vi "Get Sheet List.vi"(8 "error in (no error)":errorcluster, 11 "MS-Excel in":refnum<class "MS-Excel.lvclass">) -> (0 "error out":errorcluster, 2 "Sheet List":string[](array[string]), 3 "MS-Excel out":refnum<class "MS-Excel.lvclass">)   [LabVIEW 2017, in "LabVIEW NPOI.lvlib" / "MS-Excel.lvclass"]
doc: "Returns the names list, in <b>Sheet List</b>, of worksheets into the associated workbook to the <b>Document</b>."
uses:
  MS-Excel.lvclass
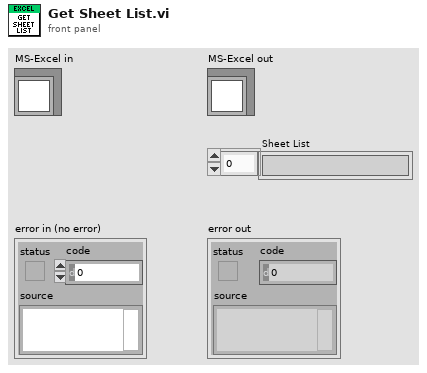
[diagram p1: front panel]
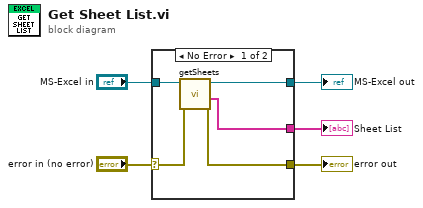
[diagram p0: block diagram]
diagram:
  n1 = case shown="No Error" "error in (no error)" {
    selector: "error in (no error)" -> [w8 w12]
    tunnel: [w7 w12] -> w4
    tunnel: [w9 w11] -> w2
    tunnel: "MS-Excel in" -> [w10 w11]
    tunnel: [w6 _] -> w1
    frame No Error {
      n2 = call-dynamic "getSheets.vi"("error in (no error)"=w8, "MS-Excel in"=w10) -> ("error out"=w7:errorcluster, "Sheet Names"=w6:string[], "MS-Excel out"=w9:refnum<class "MS-Excel.lvclass">)  [unwired: 6 in, 1 out]
    }
    frame Error {
    }
  }
  "error out" <- w4
  "MS-Excel out" <- w2
  "Sheet List" <- w1
